vi "Build Shared Library Search Path.vi"(8 "Error In":errorcluster, 11 "libssh2lv Shared Library":path=path "") -> (0 "Error Out":errorcluster, 3 "Search Path":path[](array[path]))   [LabVIEW 2021, in "Field_RnD_Services_LIBSSH2_Toolkit.lvlib" / "SSH.lvclass"]
doc: "Creates an array of paths, known as the \"Search Path\", to use to find a libssh2lv shared library."
uses:
  SSH.lvclass
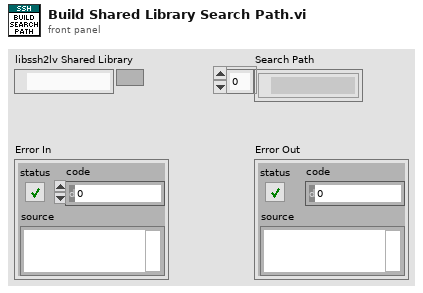
[diagram p1: front panel]
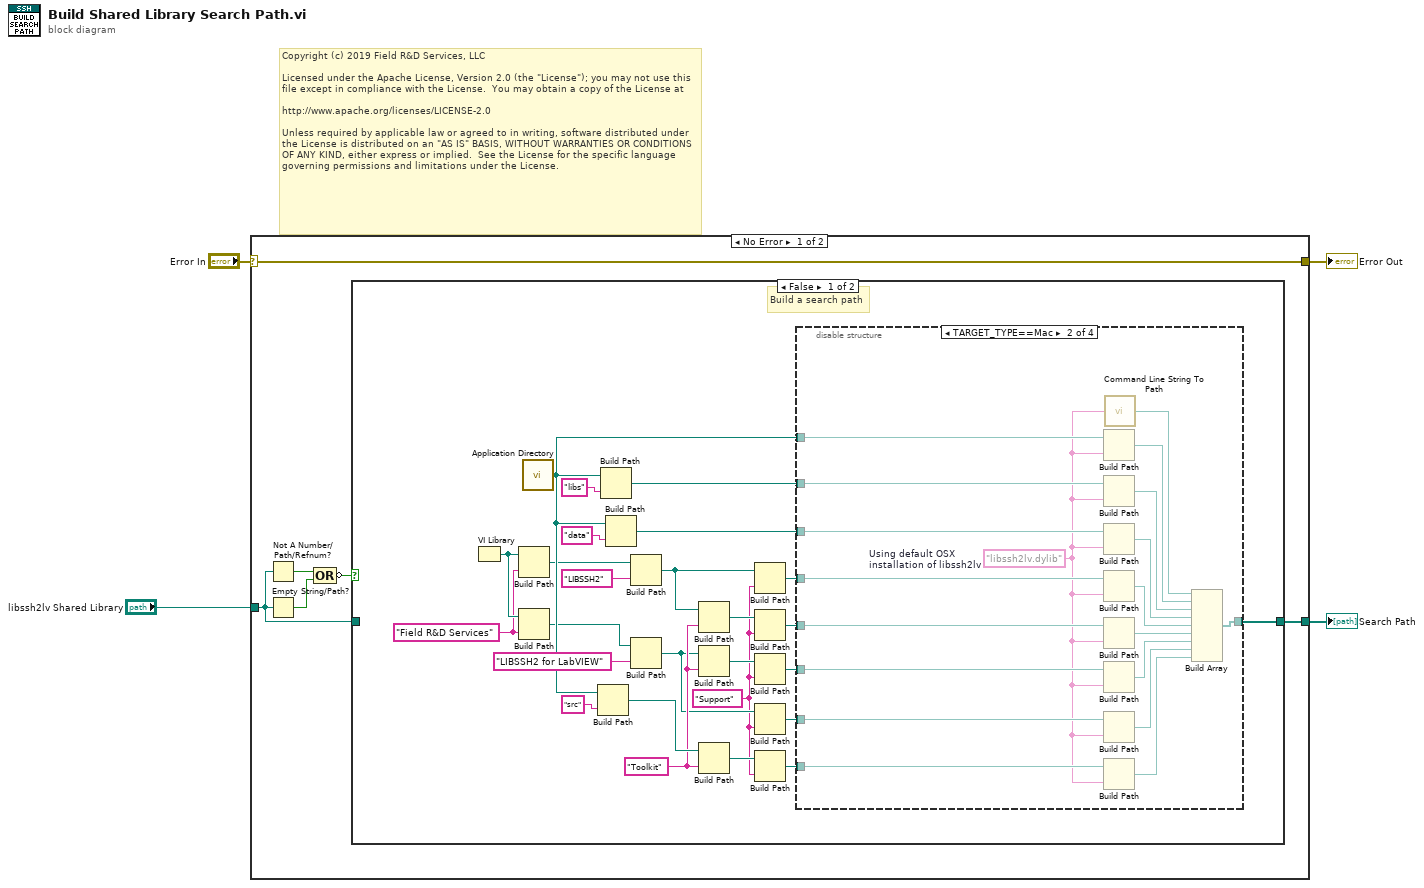
[diagram p0: block diagram]
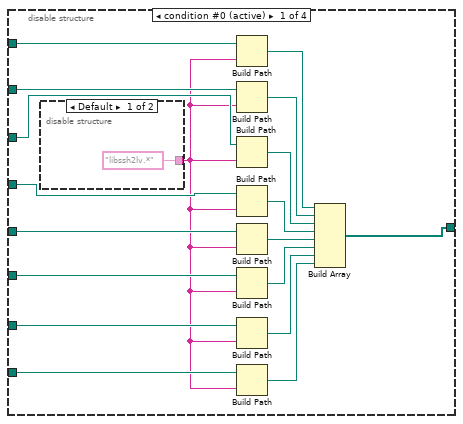
[diagram p2: hidden frame]
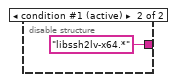
[diagram p3: hidden frame]
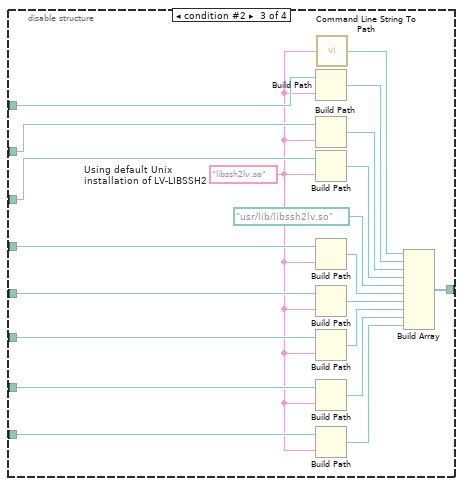
[diagram p4: hidden frame]
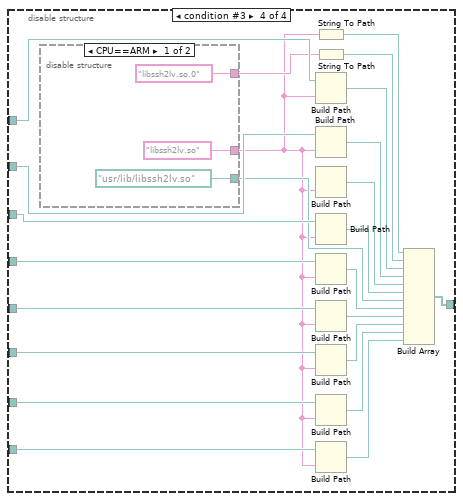
[diagram p5: hidden frame]
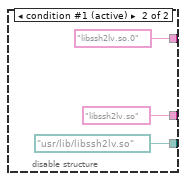
[diagram p6: hidden frame]
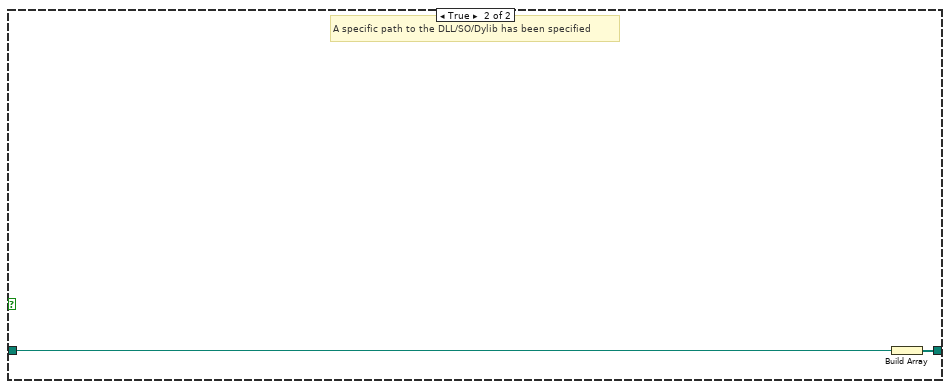
[diagram p7: hidden frame]
diagram:
  # "Copyright (c) 2019 Field R&D Services, LLC\n\nLicensed under the Apache License, Version 2.0 (the \"License\"); you may not use this file except in compliance with the License.  You may obtain a copy of the License at\n\nhttp://www.apache.org/licenses/LICENSE-2.0\n\nUnless required by applicable law or agreed to in writing, software distributed under the License is distributed on an \"AS IS\" BASIS, WITHOUT WARRANTIES OR CONDITIONS OF ANY KIND, either express or implied.  See the License for the specific language governing permissions and limitations under the License."
  n1 = case shown="No Error" "Error In" {
    selector: "Error In" -> [w9 w127]
    tunnel: [w10 _] -> w4
    tunnel: "libssh2lv Shared Library" -> [w6 _]
    tunnel: [w9 w127] -> w1
    frame No Error {
      n2 = Not A Number/Path/Refnum?(number/path/refnum=w6) -> (NaN/Path/Refnum?=w7:bool)
      n3 = Empty String/Path?(string/path=w6) -> (empty?=w8:bool)
      n4 = Compound Arithmetic op=OR(w7, w8) -> (invert w5:bool)
      n5 = case shown="False" w5 {
        tunnel: w6 -> [_ w126]
        tunnel: [w32 w125] -> w10
        frame False {
          w12 = "Support" ("name or relative path")
          w15 = "Toolkit" ("name or relative path")
          w20 = "Field R&D Services" ("name or relative path")
          # "Build a search path"
          n6 = VI Library() -> (path=w21:path)
          n7 = Build Path(base path=w21, name or relative path=w20) -> (appended path=w26:path)
          n8 = Build Path(base path=w21, name or relative path=w20) -> (appended path=w23:path)
          n9 = call <vilib>:"Application Directory.vi"() -> ("Application Directory"=w30:path)
          n10 = Build Path ("EXE include\nlocation")(base path=w30, name or relative path="src") -> (appended path=w35:path)
          n11 = Build Path ("EXE include\nlocation")(base path=w30, name or relative path="libs") -> (appended path=w27:path)
          n12 = Build Path ("EXE include\nlocation")(base path=w30, name or relative path="data") -> (appended path=w28:path)
          n13 = Build Path(base path=w26, name or relative path="LIBSSH2") -> (appended path=w18:path)
          n14 = Build Path(base path=w23, name or relative path="LIBSSH2 for LabVIEW") -> (appended path=w13:path)
          n15 = Build Path(base path=w18, name or relative path=w15) -> (appended path=w17:path)
          n16 = Build Path ("EXE include\nlocation")(base path=w13, name or relative path=w15) -> (appended path=w14:path)
          n17 = Build Path ("EXE include\nlocation")(base path=w35, name or relative path=w15) -> (appended path=w36:path)
          n18 = Build Path(base path=w18, name or relative path=w12) -> (appended path=w25:path)
          n19 = Build Path(base path=w17, name or relative path=w12) -> (appended path=w16:path)
          n20 = Build Path(base path=w14, name or relative path=w12) -> (appended path=w19:path)
          n21 = Build Path ("EXE include\nlocation")(base path=w13, name or relative path=w12) -> (appended path=w11:path)
          n22 = Build Path ("EXE include\nlocation")(base path=w36, name or relative path=w12) -> (appended path=w33:path)
          n23 = disable-structure shown="TARGET_TYPE==Mac" {
            disable-tunnel: [w53 w74 w94 w118] -> w32
            disable-tunnel: w33 -> [w54 w73 w93 w98]
            disable-tunnel: w30 -> [w52 w72 w88 w111]
            disable-tunnel: w27 -> [w51 w71 w87 w110]
            disable-tunnel: w28 -> [w50 w70 w86 w109]
            disable-tunnel: w25 -> [w49 w66 w85 w106]
            disable-tunnel: w19 -> [w42 w62 w78 w103]
            disable-tunnel: w16 -> [w43 w63 w82 w104]
            disable-tunnel: w11 -> [w41 w61 w77 w102]
            frame condition #0 (active) {
              n24 = disable-structure shown="Default" {
                disable-tunnel: ["libssh2lv.*" ("name or relative path") "libssh2lv-x64.*" ("name or relative path")] -> w40
                frame condition #0 {
                }
                frame condition #1 (active) {
                }
              }
              n25 = Build Path ("EXE include\nlocation")(base path=w52, name or relative path=w40) -> (appended path=w44:path)
              n26 = Build Path ("EXE include\nlocation")(base path=w51, name or relative path=w40) -> (appended path=w45:path)
              n27 = Build Path ("EXE include\nlocation")(base path=w50, name or relative path=w40) -> (appended path=w46:path)
              n28 = Build Path ("EXE include\nlocation")(base path=w49, name or relative path=w40) -> (appended path=w48:path)
              n29 = Build Path ("EXE include\nlocation")(base path=w43, name or relative path=w40) -> (appended path=w39:path)
              n30 = Build Path ("EXE include\nlocation")(base path=w42, name or relative path=w40) -> (appended path=w38:path)
              n31 = Build Path ("EXE include\nlocation")(base path=w41, name or relative path=w40) -> (appended path=w37:path)
              n32 = Build Path ("EXE include\nlocation")(base path=w54, name or relative path=w40) -> (appended path=w47:path)
              n33 = Build Array(w44, w45, w46, w48, w39, w38, w37, w47) -> (w53:path[])
            }
            frame condition #1 {
              w60 = "libssh2lv.dylib"  # Using default OSX installation of libssh2lv
              n34 = Build Path ("EXE include\nlocation")(base path=w72, name or relative path=w60) -> (appended path=w69:path)
              n35 = Build Path ("EXE include\nlocation")(base path=w71, name or relative path=w60) -> (appended path=w68:path)
              n36 = Build Path ("EXE include\nlocation")(base path=w70, name or relative path=w60) -> (appended path=w67:path)
              n37 = Build Path ("EXE include\nlocation")(base path=w66, name or relative path=w60) -> (appended path=w65:path)
              n38 = Build Path ("EXE include\nlocation")(base path=w63, name or relative path=w60) -> (appended path=w59:path)
              n39 = Build Path ("EXE include\nlocation")(base path=w62, name or relative path=w60) -> (appended path=w58:path)
              n40 = Build Path ("EXE include\nlocation")(base path=w61, name or relative path=w60) -> (appended path=w57:path)
              n41 = Build Path ("EXE include\nlocation")(base path=w73, name or relative path=w60) -> (appended path=w64:path)
              n42 = call <vilib>:"Command Line String To Path.vi"("string"=w60) -> ("path"=w75:path)
              n43 = Build Array(w75, w69, w68, w67, w65, w59, w58, w57, w64) -> (w74:path[])
            }
            frame condition #2 {
              w76 = "libssh2lv.so"  # Using default Unix installation of LV-LIBSSH2
              n44 = Build Path ("EXE include\nlocation")(base path=w88, name or relative path=w76) -> (appended path=w91:path)
              n45 = Build Path ("EXE include\nlocation")(base path=w87, name or relative path=w76) -> (appended path=w90:path)
              n46 = Build Path ("EXE include\nlocation")(base path=w86, name or relative path=w76) -> (appended path=w89:path)
              n47 = Build Path ("EXE include\nlocation")(base path=w85, name or relative path=w76) -> (appended path=w84:path)
              n48 = Build Path ("EXE include\nlocation")(base path=w82, name or relative path=w76) -> (appended path=w81:path)
              n49 = Build Path ("EXE include\nlocation")(base path=w78, name or relative path=w76) -> (appended path=w80:path)
              n50 = Build Path ("EXE include\nlocation")(base path=w77, name or relative path=w76) -> (appended path=w79:path)
              n51 = Build Path ("EXE include\nlocation")(base path=w93, name or relative path=w76) -> (appended path=w83:path)
              n52 = call <vilib>:"Command Line String To Path.vi"("string"=w76) -> ("path"=w95:path)
              n53 = Build Array(w95, w91, w90, w89, path "/usr/lib/libssh2lv.so" ("path"), w84, w81, w80, w79, w83) -> (w94:path[])
            }
            frame condition #3 {
              n54 = disable-structure "Conditional Disable Structure" shown="CPU==ARM" {
                disable-tunnel: ["libssh2lv.so.0" "libssh2lv.so.0"] -> w108
                disable-tunnel: ["libssh2lv.so" "libssh2lv.so"] -> w97
                disable-tunnel: [path "/usr/lib/libssh2lv.so" ("path") path "/usr/lib/libssh2lv.so" ("path")] -> w107
                frame condition #0 {
                }
                frame condition #1 (active) {
                }
              }
              n55 = String To Path(string=w97) -> (path=w117:path)
              n56 = String To Path(string=w108) -> (path=w116:path)
              n57 = Build Path ("EXE include\nlocation")(base path=w111, name or relative path=w97) -> (appended path=w112:path)
              n58 = Build Path ("EXE include\nlocation")(base path=w110, name or relative path=w97) -> (appended path=w115:path)
              n59 = Build Path ("EXE include\nlocation")(name or relative path=w97) -> (appended path=w114:path)  [unwired: 1 in]
              n60 = Build Path ("EXE include\nlocation")(base path=w109, name or relative path=w97) -> (appended path=w113:path)
              n61 = Build Path ("EXE include\nlocation")(base path=w106, name or relative path=w97) -> (appended path=w105:path)
              n62 = Build Path ("EXE include\nlocation")(base path=w104, name or relative path=w97) -> (appended path=w101:path)
              n63 = Build Path ("EXE include\nlocation")(base path=w103, name or relative path=w97) -> (appended path=w100:path)
              n64 = Build Path ("EXE include\nlocation")(base path=w102, name or relative path=w97) -> (appended path=w99:path)
              n65 = Build Path ("EXE include\nlocation")(base path=w98, name or relative path=w97) -> (appended path=w96:path)
              n66 = Build Array(w117, w116, w112, w115, w114, w113, w107, w105, w101, w100, w99, w96) -> (w118:path[])
            }
          }
        }
        frame True {
          # "A specific path to the DLL/SO/Dylib has been specified"
          n67 = Build Array(w126) -> (w125:path[])
        }
      }
    }
    frame Error {
    }
  }
  "Search Path" <- w4
  "Error Out" <- w1
